vi "PH_PPMA_PowerUnit.PC PU on.vi"(0 "i ref in":refnum<vi>, 2 "PU on":bool, 5 "error in (no error)":errorcluster) -> (14 "i ref out":refnum<vi>, 19 "error out":errorcluster)   [LabVIEW 2014, in "PH_PPMA_PowerUnit.lvlib"]
doc: "This is the action VI of the PU on event case. Depending on the inout it does the following:\n\nfalse: set save state\ntrue: if the MainAmp is not disabled and State SM = \"Stand by\", a state change request is send to SM to get \"Switch PU on\" and the attribute \"PU in use\" is set to true. \nelse: nothing is done"
uses:
  PH_PPMA_PowerUnit.lvlib
  PH_PowerUnit_BaseClass/PH_PowerUnit_BaseClass.SM States.ctl
  PH_PowerUnit_BaseClass/PH_PowerUnit_BaseClass.lvlib
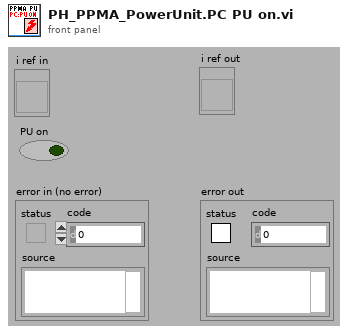
[diagram p1: front panel]
types:
  T1 = typedef "PH_PowerUnit_BaseClass.lvlib/PH_PowerUnit_BaseClass.SM States.ctl" = enum16{".", "Stand by", "Switch PU on", "Configure", "Set Default Voltage", "Set STANDBY", "Set READY", "Wait for Shot Cmd", "Open Dump Rods", "Open Ross Relais", "Close Ross Relais", "Switch PSU on", "Switch PSU off", "Charge", "Switch GD Channel on", "Close Dump Rods", "Rods-TO", "RR-TO", "PSU-TO", "Trigger-TO"}
  T2 = typedef "PH_PPMA_PowerUnit.lvlib/PH_PPMA_PowerUnit.i attribute.ctl" = cluster{"GUI Refs":cluster{"Rods":refnum<vi>, "Ignitron":refnum<vi>, "Rossrelais":refnum<vi>, "Set Voltage":refnum<vi>, "PSU":refnum<vi>, "EOC":refnum<vi>, "Trigger":refnum<vi>}, "Rods":T3, "PSU":T5, "Ross Relais":T6, "Ignitron":T7, "Trigger":cluster{"State Device":T4, "linked?":bool}, "Timing Settings":cluster{"Prdc Fast?":bool, "Default Value Periodic Interval":i32, "Mercury on since":dbl, "Warm up Time Mercury [s]":dbl}, "Set Voltage [V]":dbl}
  T3 = typedef "PH_PPMA_PowerUnit.lvlib/PH_PPMA_PowerUnit.Rods Attributes.ctl" = cluster{"Instancename":string, "Device Status":T4, "linked?":bool}
  T4 = typedef "PH_StatusHandler.lvlib/PH_StatusHandler.Status.ctl" = i16
  T5 = typedef "PH_PP_Common.lvlib/PH_PP_Common.PSU Attributes.ctl" = cluster{"lower limit [V]":dbl, "upper limit [V]":dbl, "Voltage set":bool, "State Device":T4, "linked?":bool}
  T6 = typedef "PH_PP_Common.lvlib/PH_PP_Common.Ross Relais Attributes.ctl" = cluster{"State Device":T4, "linked?":bool}
  T7 = typedef "PH_PP_Common.lvlib/PH_PP_Common.Ignitron Attributes.ctl" = cluster{"State Device":T4, "linked?":bool}
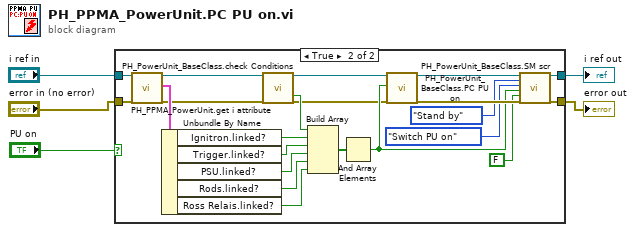
[diagram p0: block diagram]
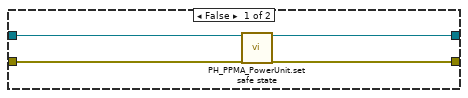
[diagram p2: hidden frame]
diagram:
  n1 = case shown="True" "PU on" {
    tunnel: "i ref in" -> [w9 w31]
    tunnel: [w8 w23] -> w5
    tunnel: "error in (no error)" -> [w7 w30]
    tunnel: [w6 w22] -> w4
    frame False {
      n2 = call "PH_PPMA_PowerUnit.set safe state.vi"("i ref in"=w9, "error in (no error)"=w7) -> ("i ref out"=w8:refnum<vi>, "error out"=w6:errorcluster)  [unwired: 16 in]
    }
    frame True {
      n3 = call "PH_PPMA_PowerUnit.get i attribute.vi"("i ref in"=w31, "error in (no error)"=w30) -> ("i ref out"=w18:refnum<vi>, "i attribute"=w29:T2, "error out"=w17:errorcluster)  [unwired: 15 in]
      n4 = Unbundle By Name(w29) -> ("Ignitron.linked?"=w27:bool, "Trigger.linked?"=w26:bool, "PSU.linked?"=w25:bool, "Rods.linked?"=w24:bool, "Ross Relais.linked?"=w15:bool)
      n5 = call "PH_PowerUnit_BaseClass.check Conditions.vi"("VI in"=w18, "error in (no error)"=w17) -> ("VI out"=w11:refnum<vi>, "Ready to switch PU on"=w16:bool, "error out"=w10:errorcluster)  [unwired: 14 in, 1 out]
      n6 = Build Array(w16, w27, w26, w25, w24, w15) -> (w28:bool[])
      n7 = And Array Elements(Boolean array=w28) -> (logical AND=w19:bool)
      n8 = call "PH_PowerUnit_BaseClass.PC PU on.vi"("i ref in"=w11, "PU on"=w19, "error in (no error)"=w10) -> ("i ref out"=w21:refnum<vi>, "error out"=w20:errorcluster)  [unwired: 15 in]
      n9 = call "PH_PowerUnit_BaseClass.SM scr.vi"("VI in"=w21, "Current SM State (condition)"=PH_PowerUnit_BaseClass.SM_States."Stand by", "Wanted SM State"=PH_PowerUnit_BaseClass.SM_States."Switch PU on", "Further change condition"=w19, "PU in use is condition? (true)"=FALSE, "error in (no error)"=w20) -> ("VI out"=w23:refnum<vi>, "error out"=w22:errorcluster)  [unwired: 12 in]
    }
  }
  "error out" <- w4
  "i ref out" <- w5
